vi "Data_folder_Path.vi"(0 "Data Type":string, 1 "FlushHierarchy":bool, 2 "SetProjectNumber":bool, 3 "ProjectNumberIn":string, 4 "Short_Name":string, 5 "seconds":dbl) -> (6 "Data Folder":path)   [LabVIEW 2015]
uses:
  Globals/Constants_global.vi
  Globals/Preference_global.vi
panel:
  out "ProjectNo":string
  out "Hierarchy":string[](array[string])
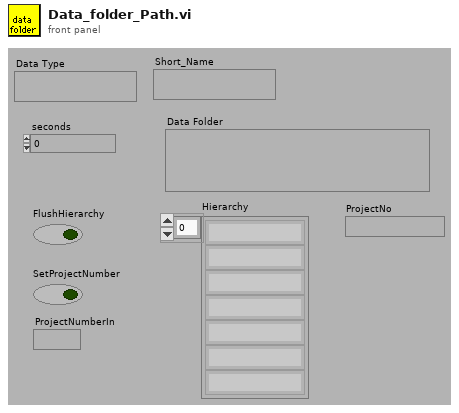
[diagram p1: front panel]
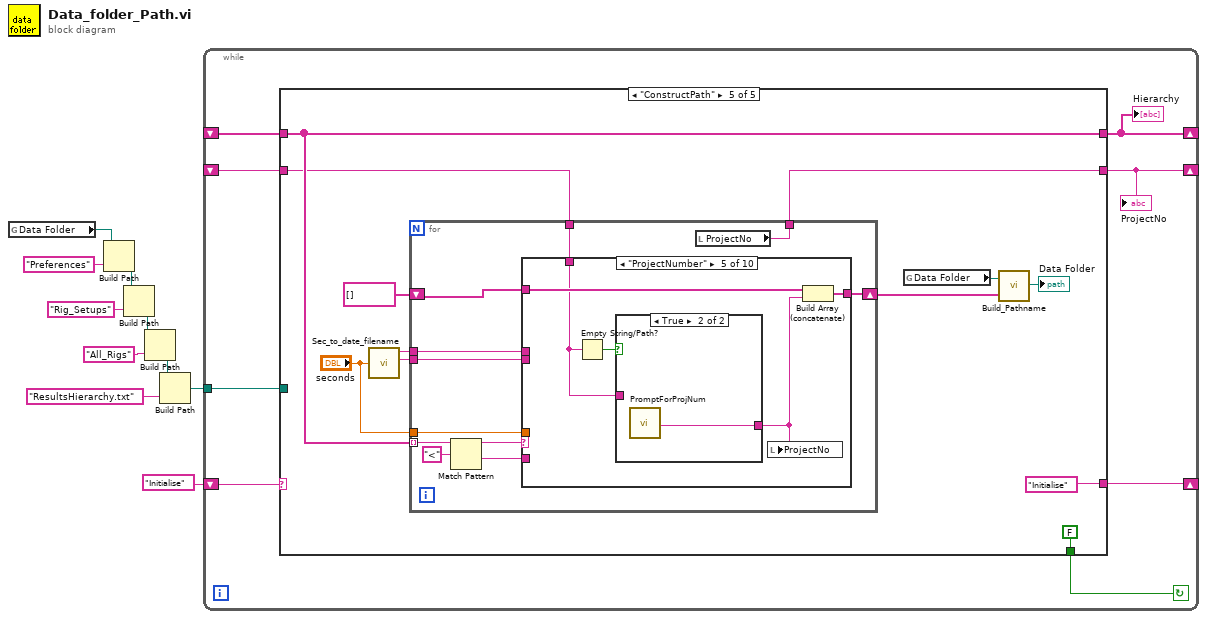
[diagram p0: block diagram]
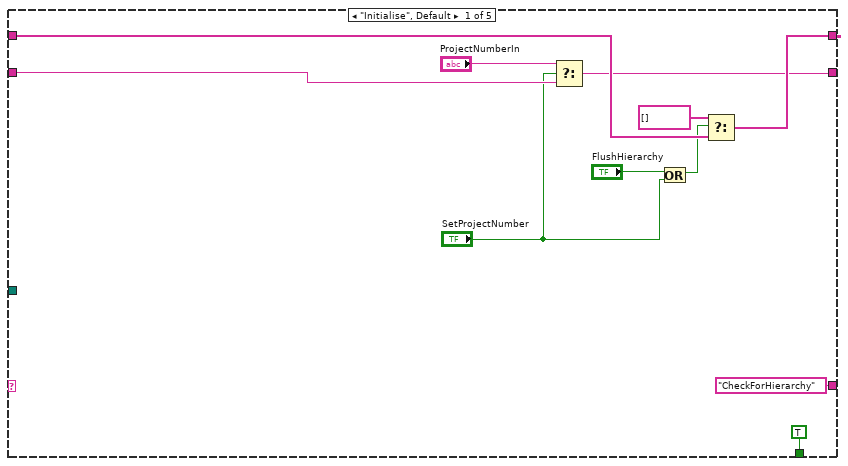
[diagram p2: hidden frame]
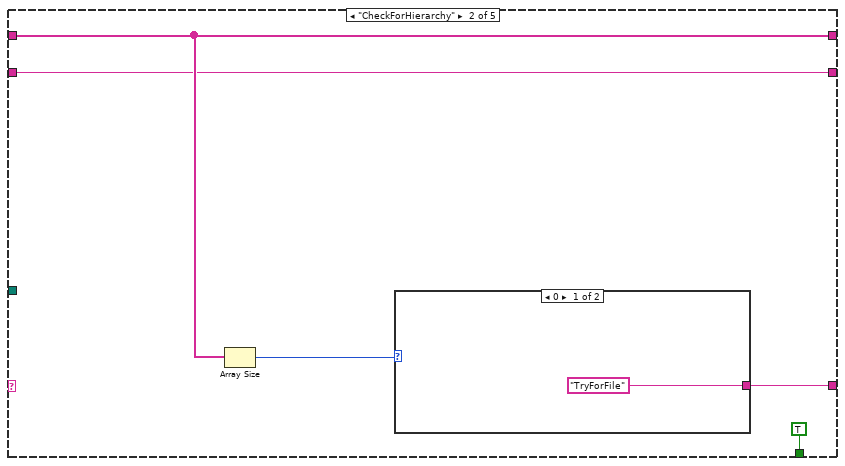
[diagram p3: hidden frame]
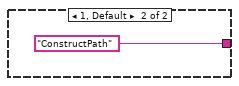
[diagram p4: hidden frame]
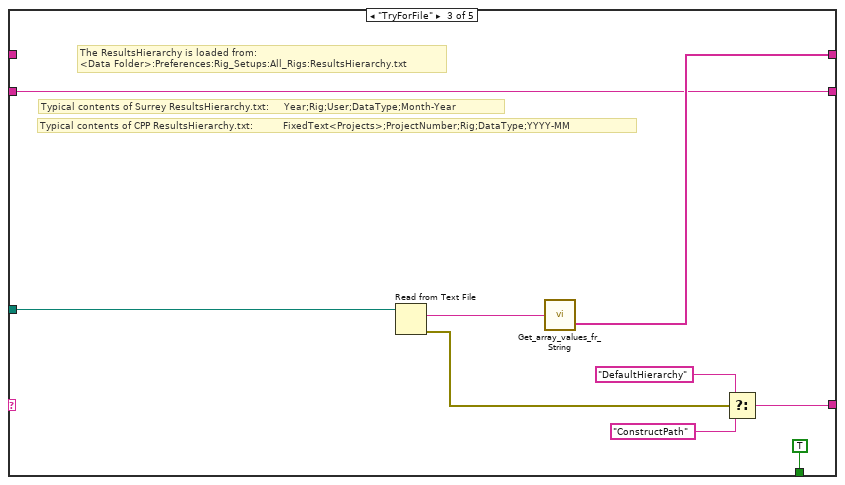
[diagram p5: hidden frame]
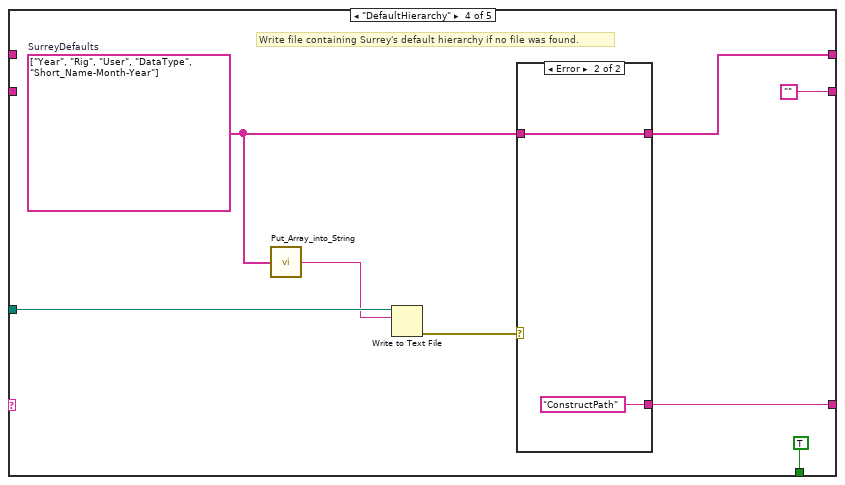
[diagram p6: hidden frame]
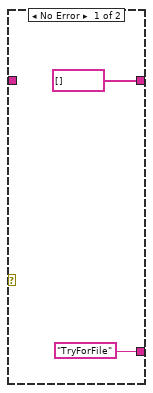
[diagram p7: hidden frame]
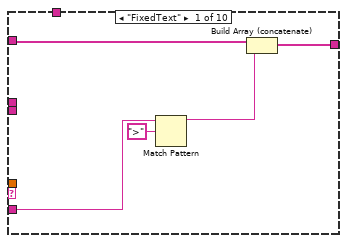
[diagram p8: hidden frame]
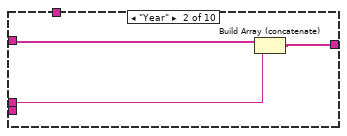
[diagram p9: hidden frame]
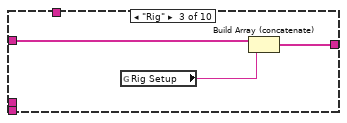
[diagram p10: hidden frame]
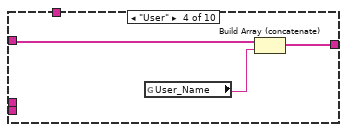
[diagram p11: hidden frame]
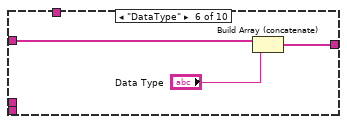
[diagram p13: hidden frame]
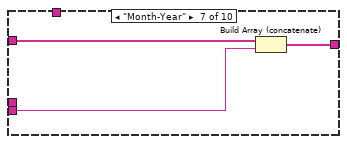
[diagram p14: hidden frame]
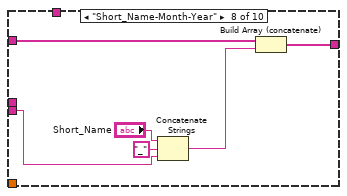
[diagram p15: hidden frame]
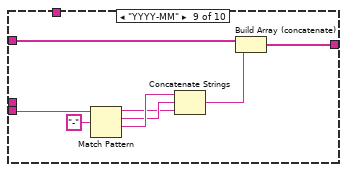
[diagram p16: hidden frame]
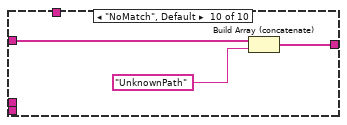
[diagram p17: hidden frame]
diagram:
  n1 = global read "Constants_global.vi" "Data Folder"() -> (w6:path)
  n2 = Build Path(base path=w6, name or relative path="Preferences") -> (appended path=w7:path)
  n3 = Build Path(base path=w7, name or relative path="Rig_Setups") -> (appended path=w8:path)
  n4 = Build Path(base path=w8, name or relative path="All_Rigs") -> (appended path=w4:path)
  n5 = Build Path(base path=w4, name or relative path="ResultsHierarchy.txt") -> (appended path=w1:path)
  n6 = while {
    shift-right: [w16] -> _
    shift-left: _ -> [w17]
    shift-right: [w15] -> _
    shift-left: "Initialise" ("t") -> [w18]
    shift-right: [w13] -> _
    shift-left: _ -> [w14]
    tunnel: w1 -> [w11]
    stop <- w12 continue-if-true
    n7 = case shown="\"ConstructPath\"" w18 {
      tunnel: w17 -> [w29 w32 _ _ w62]
      tunnel: [w28 w32 w45 w48 w62] -> w16
      tunnel: ["CheckForHierarchy" ("t") w33 w44 w46 "Initialise" ("t")] -> w15
      tunnel: w14 -> [w24 w31 w41 _ w59]
      tunnel: [w25 w31 w41 "" ("t") w58] -> w13
      tunnel: [TRUE TRUE TRUE TRUE FALSE] -> w12
      tunnel: w11 -> [_ _ w37 w51 _]
      frame "Initialise", Default {
        n8 = Select(t="ProjectNumberIn", s="SetProjectNumber", f=w24) -> (s? t:f=w25:string)
        n9 = Or(x="FlushHierarchy", y="SetProjectNumber") -> (x .or. y?=w21:bool)
        n10 = Select(t=string[] [], s=w21, f=w29) -> (s? t:f=w28:string[])
      }
      frame "CheckForHierarchy" {
        n11 = Array Size(array=w32) -> (size(s)=w34:i32)
        n12 = case shown="0" w34 {
          tunnel: ["TryForFile" ("t") "ConstructPath" ("t")] -> w33
          frame 0 {
          }
          frame 1, Default {
          }
        }
      }
      frame "TryForFile" {
        # "The ResultsHierarchy is loaded from:\n<Data Folder>:Preferences:Rig_Setups:All_Rigs:ResultsHierarchy.txt"
        # "Typical contents of CPP ResultsHierarchy.txt:          FixedText<Projects>;ProjectNumber;Rig;DataType;YYYY-MM"
        # "Typical contents of Surrey ResultsHierarchy.txt:     Year;Rig;User;DataType;Month-Year"
        n13 = Read from Text File(file (use dialog)=w37) -> (text=w39:string, error out=w38:errorcluster)  [unwired: 3 in, 2 out]
        n14 = call "Get_array_values_fr_String.vi"("String Value"=w39) -> ("String array"=w45:string[])  [unwired: 1 out]
        n15 = Select(t="DefaultHierarchy", s=w38, f="ConstructPath" ("t")) -> (s? t:f=w44:string)
      }
      frame "DefaultHierarchy" {
        w47 = string[] ["Year", "Rig", "User", "DataType", "Short_Name-Month-Year"]  # SurreyDefaults
        # "Write file containing Surrey's default hierarchy if no file was found."
        n16 = call "Put_Array_into_String.vi"("String array"=w47) -> ("String Value"=w50:string)
        n17 = Write to Text File(file (use dialog)=w51, text=w50) -> (error out=w49:errorcluster)  [unwired: 2 in, 2 out]
        n18 = case shown="Error" w49 {
          tunnel: [string[] [] ("SurreyDefaults") w57] -> w48
          tunnel: w47 -> [_ w57]
          tunnel: ["TryForFile" ("t") "ConstructPath" ("t")] -> w46
          frame No Error {
          }
          frame Error {
          }
        }
      }
      frame "ConstructPath" {
        n19 = call "Sec_to_date_filename.vi"("seconds"="seconds") -> ("Year"=w67:string, "Month"=w66:string)  [unwired: 2 out]
        n20 = for {
          shift-right: [w80] -> w65
          shift-left: string[] [] -> [w79]
          tunnel: w62 -> [w75] mode=indexing
          tunnel: w66 -> [w78]
          tunnel: w67 -> [w77]
          tunnel: "seconds" -> [w76]
          tunnel: w59 -> [w71]
          tunnel: [w70] -> w58
          n21 = Match Pattern(string=w75, regular expression="<") -> (before substring=w74:string, after substring=w72:string)  [unwired: 1 in, 2 out]
          n22 = case shown="\"ProjectNumber\"" w74 {
            tunnel: [w85 w88 w90 w94 w99 w104 w107 w113 w119 w124] -> w80
            tunnel: w79 -> [w84 w87 w89 w92 w98 w103 w106 w112 w118 w123]
            tunnel: w78 -> [_ _ _ _ _ _ w105 w109 w121 _]
            tunnel: w77 -> [_ w86 _ _ _ _ _ _ _ _]
            tunnel: w76 -> [_ _ _ _ _ _ _ _ _ _]
            tunnel: w72 -> [w83 _ _ _ _ _ _ _ _ _]
            tunnel: w71 -> [_ _ _ _ w96 _ _ _ _ _]
            frame "FixedText" {
              n23 = Match Pattern(string=w83, regular expression=">") -> (before substring=w81:string)  [unwired: 1 in, 3 out]
              n24 = Build Array (concatenate)(w84, w81) -> (w85:string[])
            }
            frame "Year" {
              n25 = Build Array (concatenate)(w87, w86) -> (w88:string[])
            }
            frame "Rig" {
              n26 = global read "Preference_global.vi" "Rig Setup"() -> (w91:string)
              n27 = Build Array (concatenate)(w89, w91) -> (w90:string[])
            }
            frame "User" {
              n28 = global read "Preference_global.vi" "User_Name"() -> (w93:string)
              n29 = Build Array (concatenate)(w92, w93) -> (w94:string[])
            }
            frame "ProjectNumber" {
              n30 = Empty String/Path?(string/path=w96) -> (empty?=w97:bool)
              n31 = case shown="True" w97 {
                tunnel: [w100 w101] -> w95
                tunnel: w96 -> [w100 _]
                frame False {
                }
                frame True {
                  n32 = call "PromptForProjNum.vi"() -> ("ProjectNumber"=w101:string)  [unwired: 17 in, 2 out]
                }
              }
              n33 = local write "ProjectNo"(w95) -> ()
              n34 = Build Array (concatenate)(w98, w95) -> (w99:string[])
            }
            frame "DataType" {
              n35 = Build Array (concatenate)(w103, "Data Type") -> (w104:string[])
            }
            frame "Month-Year" {
              n36 = Build Array (concatenate)(w106, w105) -> (w107:string[])
            }
            frame "Short_Name-Month-Year" {
              n37 = Concatenate Strings("Short_Name", "_" ("string"), w109) -> (w108:string)
              n38 = Build Array (concatenate)(w112, w108) -> (w113:string[])
            }
            frame "YYYY-MM" {
              n39 = Match Pattern(string=w121, regular expression="-") -> (before substring=w115:string, match substring=w116:string, after substring=w117:string)  [unwired: 1 in, 1 out]
              n40 = Concatenate Strings(w117, w116, w115) -> (w114:string)
              n41 = Build Array (concatenate)(w118, w114) -> (w119:string[])
            }
            frame "NoMatch", Default {
              n42 = Build Array (concatenate)(w123, "UnknownPath" ("element")) -> (w124:string[])
            }
          }
          n43 = local read "ProjectNo"() -> (w70:string)
        }
        n44 = global read "Constants_global.vi" "Data Folder"() -> (w63:path)
        n45 = call "Build_Pathname.vi"("PathElements"=w65, "PathnameIn"=w63) -> ("AppendedPath"=→"Data Folder":path)
      }
    }
    "Hierarchy" <- w16
    "ProjectNo" <- w13
  }
